vi "PathInit.vi"(0 "基路径":path) -> ()   [LabVIEW 2014]
uses:
  Global.vi
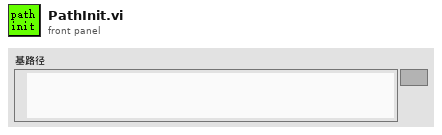
[diagram p1: front panel]
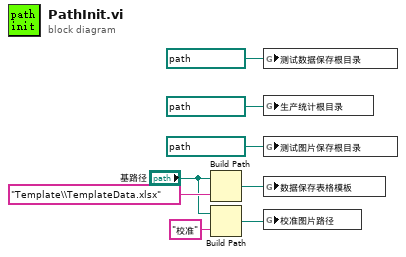
[diagram p0: block diagram]
diagram:
  n1 = Build Path(base path="基路径", name or relative path="Template\\TemplateData.xlsx" ("名称或相对路径")) -> (appended path=w5:path)
  n2 = Build Path(base path="基路径", name or relative path="校准" ("名称或相对路径")) -> (appended path=w1:path)
  n3 = global write "Global.vi" "测试数据保存根目录"(path "D:/测试数据" ("Cam1ImgSaveFoldPath")) -> ()
  n4 = global write "Global.vi" "生产统计根目录"(path "D:/生产统计" ("Cam1ImgSaveFoldPath")) -> ()
  n5 = global write "Global.vi" "测试图片保存根目录"(path "D:/测试图片" ("Cam1ImgSaveFoldPath")) -> ()
  n6 = global write "Global.vi" "数据保存表格模板"(w5) -> ()
  n7 = global write "Global.vi" "校准图片路径"(w1) -> ()
